vi "DataProcess.vi"(8 "error in (no error)":errorcluster) -> (0 "error out":errorcluster)   [LabVIEW 2016]
uses:
  <vilib>/Platform/TimedLoop/XDataNode/timing_clust.ctl
  <vilib>/Platform/TimedLoop/XDataNode/nitl_modes.ctl
  <vilib>/Platform/TimedLoop/XDataNode/wakeup.ctl
  Typedef/Filter Data.ctl
  Typedef/INS Data.ctl
  <vilib>/Analysis/coordinate.llb/Wrap Angle (scalar).vi
  <vilib>/platform/TimedLoop/XDataNode/XDataNode.xnode
  <vilib>/Platform/TimedLoop/XDataNode/XDNodeRunTimeDep.lvlib
  <vilib>/ptbypt/NI_PtbyPt.lvlib
  <vilib>/Analysis/NI_AAL_Angle.lvlib
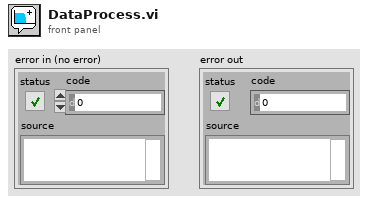
[diagram p1: front panel]
types:
  T1 = typedef "XDNodeRunTimeDep.lvlib/timing_clust.ctl" = cluster{"Expected End [f-1]":u64, "Actual End [f-1]":u64, "Finished Late? [f-1]":bool, "Expected End [i-1]":u64, "Actual End [i-1]":u64, "Finished Late? [i-1]":bool, "Expected Start [i]":u64, "Actual Start [i]":u64, "Expected Start [f]":u64, "Actual Start [f]":u64, "Source Name":string, "Structure Name":string, "Period":i64, "Deadline":i64, "Offset":i64, "Start":i64, "Priority":i32, "Timeout":i32, "Mode":T2, "Wakeup Reason":T3, "Error":errorcluster, "Source Type":string, "Secondary Source Type":string, "Global End Time":u64, "Global Start Time":u64, "Frame Duration":u64, "Iteration Duration":u64, "Assigned CPU":i32, "I/O Scan Engine Mode":u32}
  T2 = typedef "XDNodeRunTimeDep.lvlib/nitl_modes.ctl" = enum32{"No Change", "Process missed periods, maintain original phase", "Discard missed periods, maintain original phase", "Process missed periods, ignore original phase", "Discard missed periods, ignore original phase"}
  T3 = typedef "XDNodeRunTimeDep.lvlib/wakeup.ctl" = enum32{"Normal", "Aborted", "Asynchronous wakeup", "Timing source error", "Timed loop error", "Timeout"}
  T4 = typedef "Filter Data.ctl" = cluster{"Yaw":dbl, "Lat":dbl, "Long":dbl}
  T5 = typedef "INS Data.ctl" = cluster{"Yaw":sgl, "Pitch":sgl, "Roll":sgl, "Lat":dbl, "Long":dbl, "Alt":dbl, "North":dbl, "East":dbl, "Down":dbl, "PosU":dbl, "VelU":dbl}
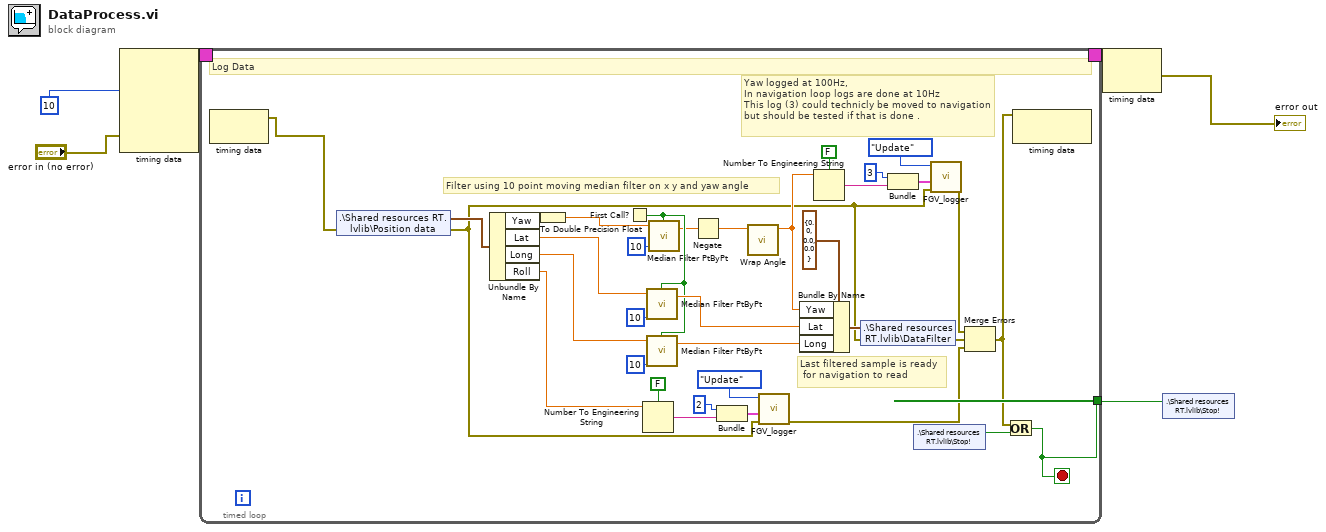
[diagram p0: block diagram]
diagram:
  n1 = node-c288(i64 10 ("Period"), "error in (no error)") -> (w5:T1)  [unwired: 3 in]
  n2 = timed-loop {
    tunnel: [w41] -> w6
    timing: w5 -> [_]
    timing-out: [_] -> w4
    stop <- w41 stop-if-true
    # "Last filtered sample is ready\n for navigation to read"
    # "Yaw logged at 100Hz, \nIn navigation loop logs are done at 10Hz\nThis log (3) could technicly be moved to navigation but should be tested if that is done ."
    # "Filter using 10 point moving median filter on x y and yaw angle"
    # "Log Data"
    n3 = node-c288() -> (w39:errorcluster)  [unwired: 1 in]
    n4 = shared-variable ".\\Shared resources RT.lvlib\\Position data"(error in=w39) -> (w38:T5, error out=w8:errorcluster)
    n5 = Unbundle By Name(w38) -> ("Yaw"=w37:sgl, "Lat"=w29:dbl, "Long"=w28:dbl, "Roll"=w12:sgl)
    n6 = To Double Precision Float(number=w37) -> (double precision float=w35:dbl)
    n7 = First Call?() -> (First Call?: T/F=w25:bool)
    n8 = Number To Engineering String(1:FALSE ("use system decimal point (T)"), 4:w12) -> (0:w16:string)  [unwired: 2 in]
    n9 = call <vilib>:"Median Filter PtByPt.vi"("initialize"=w25, "rank"=10, "x"=w29) -> ("Filtered x"=w27:dbl)  [unwired: 1 in, 1 out]
    n10 = call <vilib>:"Median Filter PtByPt.vi"("initialize"=w25, "rank"=10, "x"=w28) -> ("Filtered x"=w26:dbl)  [unwired: 1 in, 1 out]
    n11 = call <vilib>:"Median Filter PtByPt.vi"("initialize"=w25, "rank"=10, "x"=w35) -> ("Filtered x"=w19:dbl)  [unwired: 1 in, 1 out]
    n12 = Negate(x=w19) -> (-x=w9:dbl)
    n13 = Bundle(2, w16) -> (w17:cluster{i32, string})  [unwired: 1 in]
    n14 = call-poly <vilib>:"Wrap Angle.vi"("angle in"=w9) -> ("angle out"=w18:dbl)  [unwired: 9 in, 1 out]
    n15 = call "FGV_logger.vi"("error in"=w8, 9:w17, "Command"=enum16{"Update", "Log", "Init"}."Update") -> ("error out"=w10:errorcluster)  [unwired: 8 in]
    n16 = Bundle By Name(cluster=T4 {"Yaw"=0.0, "Lat"=0.0, "Long"=0.0} ("Filter Data"), "Yaw"=w18, "Lat"=w27, "Long"=w26) -> (w32:T4)
    n17 = Number To Engineering String(1:FALSE ("use system decimal point (T)"), 4:w18) -> (0:w23:string)  [unwired: 2 in]
    n18 = shared-variable ".\\Shared resources RT.lvlib\\DataFilter"(w32, error in=w8) -> (error out=w11:errorcluster)
    n19 = Bundle(3, w23) -> (w24:cluster{i32, string})  [unwired: 1 in]
    n20 = shared-variable ".\\Shared resources RT.lvlib\\Stop!"() -> (w36:bool)  [unwired: 1 in, 1 out]
    n21 = call "FGV_logger.vi"("error in"=w8, 9:w24, "Command"=enum16{"Update", "Log", "Init"}."Update") -> ("error out"=w7:errorcluster)  [unwired: 8 in]
    n22 = Merge Errors(w7, w11, w10) -> (w40:errorcluster)
    n23 = Or(x=w40, y=w36) -> (x .or. y?=w41:bool)
    n24 = node-c288(w40) -> ()  [unwired: 1 out]
  }
  n25 = node-c288(w4) -> (→"error out":errorcluster)
  n26 = shared-variable ".\\Shared resources RT.lvlib\\Stop!"(w6) -> ()  [unwired: 1 in, 1 out]
